vi "Write to Max Min frame global.vi"(9 "Max cursor / End frame":i32, 11 "Min cursor / Start frame":i32) -> ()   [LabVIEW 2013]
uses:
  Globals/gl_Time series viewer globals.vi
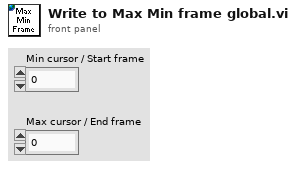
[diagram p1: front panel]
types:
  T1 = cluster{"Start Frame No":i32, "End Frame No":i32}
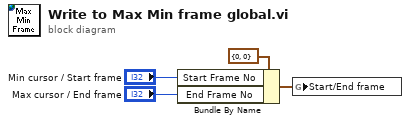
[diagram p0: block diagram]
diagram:
  n1 = Bundle By Name(cluster=T1 {"Start Frame No"=0, "End Frame No"=0} ("Video Frame"), "Start Frame No"="Min cursor / Start frame", "End Frame No"="Max cursor / End frame") -> (w1:T1)
  n2 = global write "gl_Time series viewer globals.vi" "Start/End frame"(w1) -> ()
